vi "Ensure Filename Has Extension.vi"(1 "Desired File Extension":T1, 2 "Filename (with or without extension)":string) -> (0 "Filename With Extension":string)   [LabVIEW 2022 SP3]
doc: "<add documentation here>"
uses:
  Output File Extension (enum).ctl
panel:
  # "Development\nControls or indicators that are useful for development or testing, but which are not outputs of the VI."
  # "Input\nInputs to the VI"
  # "Output\nOutputs of the VI"
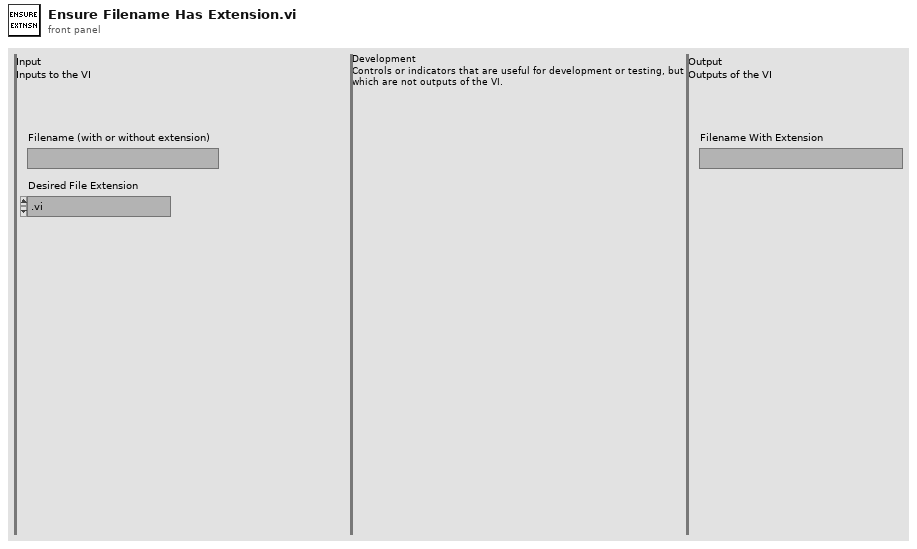
[diagram p1: front panel]
types:
  T1 = typedef "Output File Extension (enum).ctl" = enum16{".vi", ".ctl"}
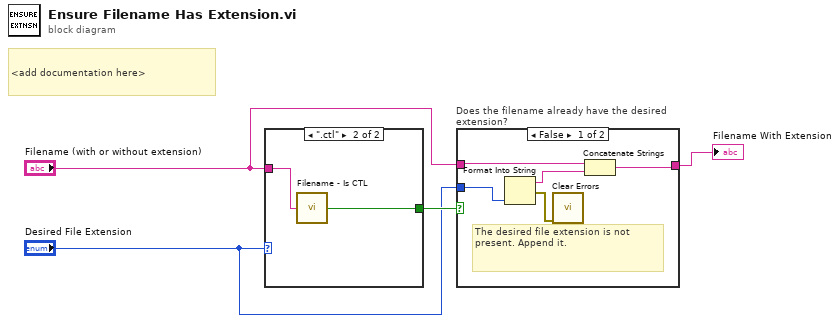
[diagram p0: block diagram]
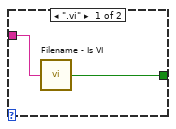
[diagram p3: hidden frame]
diagram:
  # "<add documentation here>"
  n1 = case shown="\".ctl\"" "Desired File Extension" {
    tunnel: "Filename (with or without extension)" -> [w6 w8]
    tunnel: [w5 w7] -> w4
    frame ".vi" {
      n2 = call "Filename - Is VI.vi"("Filename (including file extension)"=w6) -> ("Is VI?"=w5:bool)
    }
    frame ".ctl" {
      n3 = call "Filename - Is CTL.vi"("Filename (including file extension)"=w8) -> ("Is CTL?"=w7:bool)
    }
  }
  n4 = case "Does the filename already have the desired extension?" shown="False" w4 {
    tunnel: "Filename (with or without extension)" -> [w13 w14]
    tunnel: [w9 w14] -> w2
    tunnel: "Desired File Extension" -> [w12 _]
    frame False {
      # "The desired file extension is not present. Append it."
      n5 = Format Into String(w12) -> (resulting string=w11:string, error out=w10:errorcluster)  [unwired: 3 in]
      n6 = call <vilib>:"Clear Errors.vi"("error in (no error)"=w10) -> ()  [unwired: 5 in, 2 out]
      n7 = Concatenate Strings(w13, w11) -> (w9:string)
    }
    frame True {
      # "The desired file extension is already present. No need to modify."
    }
  }
  "Filename With Extension" <- w2
